vi "Write_USB.vi"(8 "entrée d'erreur":errorcluster caption="entrée d'erreur (pas d'erreur)", 10 "buffer d'écriture":string, 11 "Nom de ressource VISA":refnum<visa-resource-name>) -> (0 "sortie d'erreur":errorcluster, 3 "Nom de ressource VISA en sortie":refnum<visa-resource-name>)   [LabVIEW 2014]
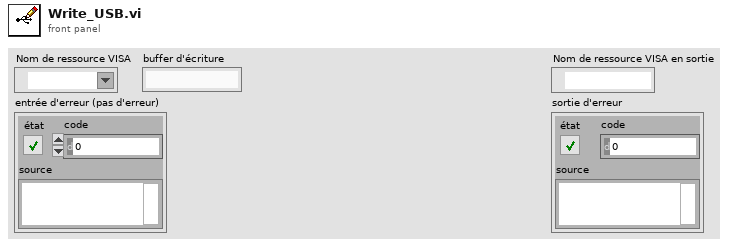
[diagram p1: front panel]
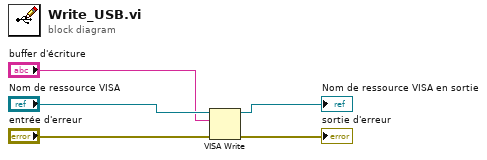
[diagram p0: block diagram]
diagram:
  n1 = VISA Write(VISA resource name="Nom de ressource VISA", write buffer="buffer d'écriture", error in (no error)="entrée d'erreur") -> (VISA resource name out=→"Nom de ressource VISA en sortie":refnum<visa-resource-name>, error out=→"sortie d'erreur":errorcluster)  [unwired: 1 out]
